vi "ActionVIOnCompile.vi"(8 "error in (no error)":errorcluster, 11 "Device Item Ref in":T1 format="%.0x") -> (0 "error out":errorcluster)   [LabVIEW 2019, in "MD4Logger System Explorer.lvlib"]
uses:
  <vilib>/NI VeriStand/Custom Device API/Custom Device Item Ref.ctl
  <vilib>/NI VeriStand/Custom Device Tools/Custom Device Utility Library/NI VeriStand - Search for Item by Name.vi
  <vilib>/NI VeriStand/Custom Device API/Set Item Property (Variant).vi
  MD4Logger System Explorer.lvlib
  <vilib>/NI VeriStand/Custom Device Tools/Custom Device Utility Library/Custom Device Utility Library.lvlib
  <vilib>/NI VeriStand/Custom Device API/Custom Device API.lvlib
  <vilib>/NI/NIVS Inline Async API/_Data Access System Explorer/Data Access System Explorer.lvlib
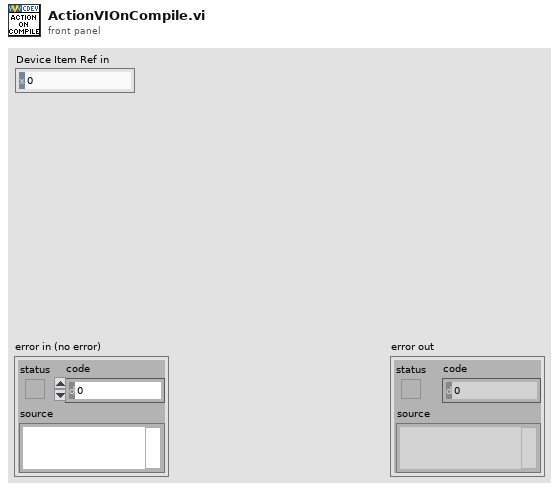
[diagram p1: front panel]
types:
  T1 = typedef "Custom Device API.lvlib/Custom Device Item Ref.ctl" = u64
  T2 = cluster{"Name":string, "Type":enum16{"Output/Write", "Input/Read", "Input/ReadWrite"}, "VS Refs":T1[]}
  T3 = enum16{"Output/Write", "Input/Read", "Input/ReadWrite"}
  T4 = typedef "Custom Device API.lvlib/Custom Device Item Info.ctl" = cluster{"Name":string, "Is Channel":bool, "GUID":string, "Is Waveform":bool}
  T5 = cluster{"Name":string, "Type":enum16{"Output/Write", "Input/Read", "Input/ReadWrite"}, "VS Refs":T1[]}[]
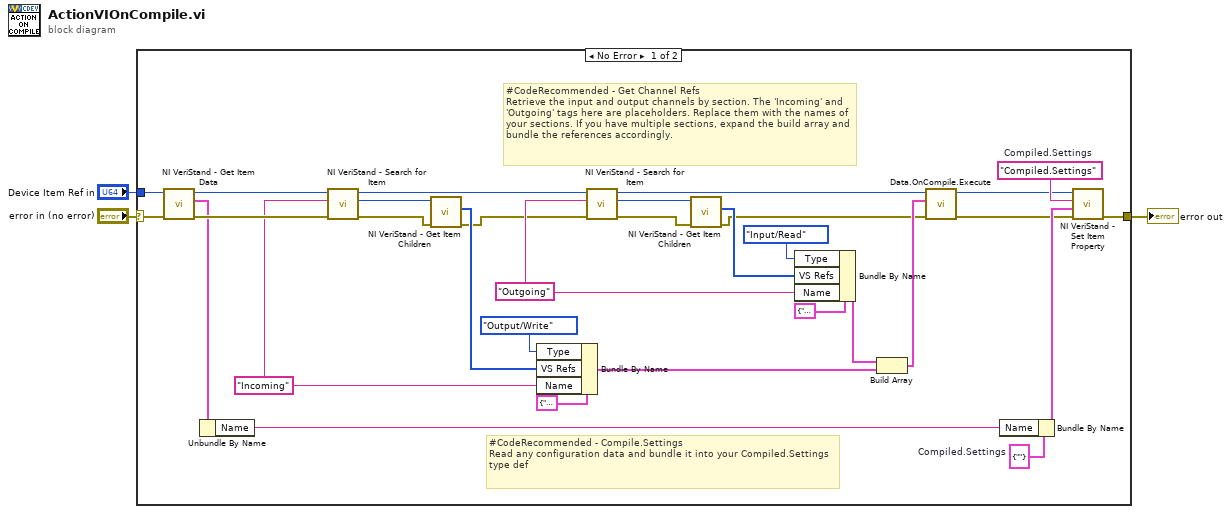
[diagram p0: block diagram]
diagram:
  n1 = case shown="No Error" "error in (no error)" {
    selector: "error in (no error)" -> [w27 w35]
    tunnel: [w28 w35] -> w2
    tunnel: "Device Item Ref in" -> [w26 _]
    frame No Error {
      w4 = cluster{"Name":string} {"Name"=""}  # Compiled.Settings
      w19 = "Outgoing" ("Item Name")
      w21 = "Incoming" ("Item Name")
      w30 = "Compiled.Settings"  # Compiled.Settings
      # "#CodeRecommended - Get Channel Refs\nRetrieve the input and output channels by section. The 'Incoming' and 'Outgoing' tags here are placeholders. Replace them with the names of your sections. If you have multiple sections, expand the build array and bundle the references accordingly."
      # "#CodeRecommended - Compile.Settings\nRead any configuration data and bundle it into your Compiled.Settings type def"
      n2 = call <vilib>:"NI VeriStand - Get Item Data.vi"("error in (no error)"=w27, "Item Ref in"=w26) -> ("error out"=w24:errorcluster, "Item Info"=w23:T4, "Item Ref out"=w25:T1)  [unwired: 6 in, 1 out]
      n3 = Unbundle By Name(w23) -> ("Name"=w22:string)
      n4 = call-poly <vilib>:"NI VeriStand - Search for Item.vi"("error in"=w24, "Item Name"=w21, "Section Ref in"=w25) -> ("error out"=w34:errorcluster, "Item Ref"=w33:T1, "Section Ref out"=w8:T1)  [unwired: 5 in, 1 out]
      n5 = call <vilib>:"NI VeriStand - Get Item Children.vi"("error in (no error)"=w34, "Item Ref in"=w33) -> ("error out"=w7:errorcluster, "Child Refs"=w20:T1[])  [unwired: 6 in, 2 out]
      n6 = Bundle By Name(cluster=T2 {"Name"="", "Type"=enum."Output/Write", "VS Refs"=[]} ("Group"), "Type"=T3."Output/Write", "VS Refs"=w20, "Name"=w21) -> (w11:T2)
      n7 = call-poly <vilib>:"NI VeriStand - Search for Item.vi"("error in"=w7, "Item Name"=w19, "Section Ref in"=w8) -> ("error out"=w31:errorcluster, "Item Ref"=w32:T1, "Section Ref out"=w9:T1)  [unwired: 5 in, 1 out]
      n8 = call <vilib>:"NI VeriStand - Get Item Children.vi"("error in (no error)"=w31, "Item Ref in"=w32) -> ("error out"=w10:errorcluster, "Child Refs"=w15:T1[])  [unwired: 6 in, 2 out]
      n9 = Bundle By Name(cluster=T2 {"Name"="", "Type"=enum."Output/Write", "VS Refs"=[]} ("Group"), "Type"=T3."Input/Read", "VS Refs"=w15, "Name"=w19) -> (w17:T2)
      n10 = Build Array(w17, w11) -> (w14:T5)
      n11 = call <vilib>:"Data.OnCompile.Execute.vi"("error in"=w10, "VS Ref Groups"=w14, "Custom Device Ref"=w9) -> ("error out"=w6:errorcluster, "Custom Device Ref"=w5:T1)  [unwired: 7 in]
      n12 = Bundle By Name(cluster=w4, "Name"=w22) -> (w29:cluster{"Name":string})
      n13 = call-poly <vilib>:"NI VeriStand - Set Item Property.vi"("error in (no error)"=w6, "Value"=w29, "Property Name"=w30, "Item Ref in"=w5) -> ("error out"=w28:errorcluster)  [unwired: 5 in, 2 out]
    }
    frame Error {
    }
  }
  "error out" <- w2
